vi "SLL DE AI Channel Unit Infomation.vi"(8 "error in (no error)":errorcluster) -> (0 "error out":errorcluster, 3 "Unit Infomation":T2(array[cluster]))   [LabVIEW 2013]
doc: "Copyright © 2005, Soliton Technologies.\nAll rights reserved."
uses:
  Controls/SLL DE DAQ Parameters LV2Global Options.ctl
  Controls/SLL DE List of AI Channel Type.ctl
  Controls/SLL DE Unit Info LV2Global Options.ctl
panel:
  in  "Channel Type":T1
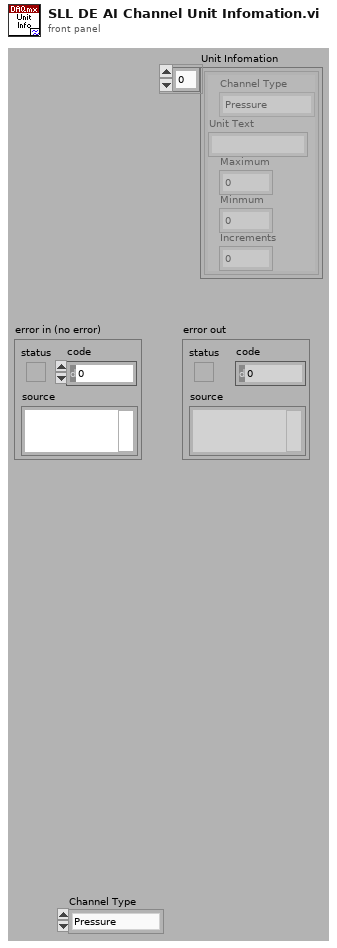
[diagram p1: front panel]
types:
  T1 = typedef "SLL DE List of AI Channel Type.ctl" = enum16{"Pressure", "Flow", "Temperature", "Time Scale", "Voltage", "Current", "Frequency", "Sound", "Speed", "Torque", "Distance", "Channel Type 1", "Channel Type 2", "Channel Type 3"}
  T2 = cluster{"Channel Type":T1, "Unit Text":string, "Maximum":dbl, "Minmum":dbl, "Increments":dbl}[]
  T3 = typedef "SLL DE Unit Info LV2Global Options.ctl" = enum16{"Update Channel Type", "Update Unit Info", "Get Unit Info", "Read"}
  T4 = typedef "SLL DE DAQ Parameters LV2Global Options.ctl" = enum16{"Read", "Write"}
  T5 = typedef "SLL DE DAQ Engine Parameters.ctl" = cluster{"Enable Engines":cluster{"AI Enable":bool, "AO Enable":bool, "DI Enable":bool, "DO Enable":bool}, "DAQ Control Type":cluster{"Analog Input":enum16{"Finite", "Continuous", "Driver"}, "Analog Output":enum16{"Finite", "Continuous", "Driver"}, "Digital Input":enum16{"Finite", "Continuous", "Driver"}, "Digital Output":enum16{"Finite", "Continuous", "Driver"}}, "DAQ Parameters":cluster{"AI Sampling Rate (Samples/Sec)":dbl, "MvgAVG Window Size (# of Points)":i32, "Enable Filter":bool, "Enable MvgAVG":bool, "Circular Buffer Size (Sec)":dbl, "AO Sampling Rate (Samples/Sec)":dbl, "Graph Update Rate (Samples/Sec)":dbl, "File Logging Rate (Samples/Sec)":i32}, "AO Safe Values":cluster{"Analog Outputs Name":T6, "Analog Outputs Safe Value":dbl}[], "DO Safe Values":cluster{"Digital Outputs Name":T7, "Digital Outputs Safe Value":bool}[], "DO Interconnected Lines":cluster{"First DO Line":string, "Second DO Line":string}[], "AI Channels Unit":cluster{"Channel Name":T8, "Channel Type":T1}[], "Units Information":cluster{"Channel Type":T1, "Unit Text":string, "Maximum":dbl, "Minmum":dbl, "Increments":dbl}[]}
  T6 = typedef "SLL DE List of Analog Outputs.ctl" = enum16{"None"}
  T7 = typedef "SLL DE List of Digital Outputs.ctl" = enum16{"STATION1_START TEST", "STATION1_STOP TEST", "STATION1_LIGHT1", "STATION1_LIGHT2", "STATION1_LIGHT3", "STATION1_SELECT_TEST", "STATION2_START TEST", "STATION2_STOP TEST", "STATION2_LIGHT1", "STATION2_LIGHT2", "STATION2_LIGHT3", "STATION2_SELECT_TEST", "STATION3_START TEST", "STATION3_STOP TEST", "STATION3_LIGHT1", "STATION3_LIGHT2", "STATION3_LIGHT3", "STATION3_SELECT_TEST", "STATION4_START TEST", "STATION4_STOP TEST", "STATION4_LIGHT1", "STATION4_LIGHT2", "STATION4_LIGHT3", "STATION4_SELECT_TEST"}
  T8 = typedef "SLL DE List of Analog Inputs.ctl" = enum16{"None"}
  T9 = cluster{"Channel Type":T1, "Unit Text":string, "Maximum":dbl, "Minmum":dbl, "Increments":dbl}
  T10 = cluster{"Channel Type":T1, string, "Maximum":dbl, "Minmum":dbl, "Increments":dbl}
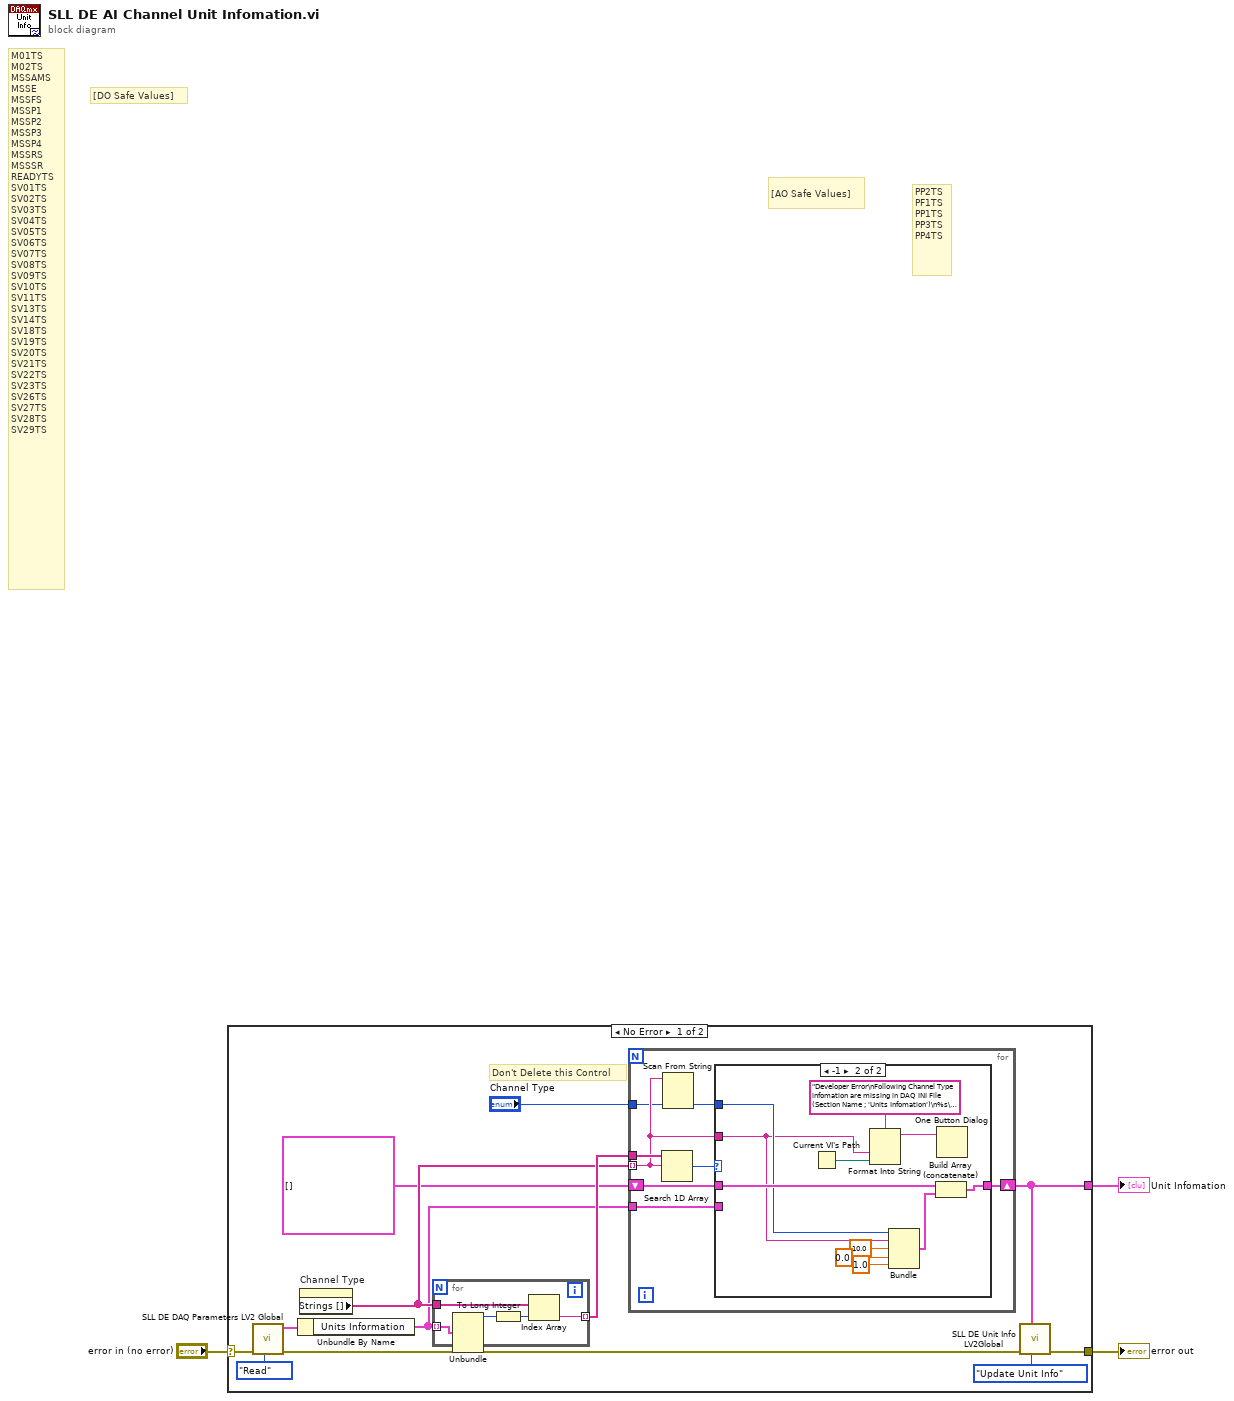
[diagram p0: block diagram]
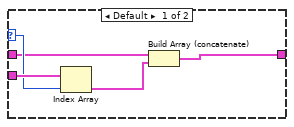
[diagram p2: hidden frame]
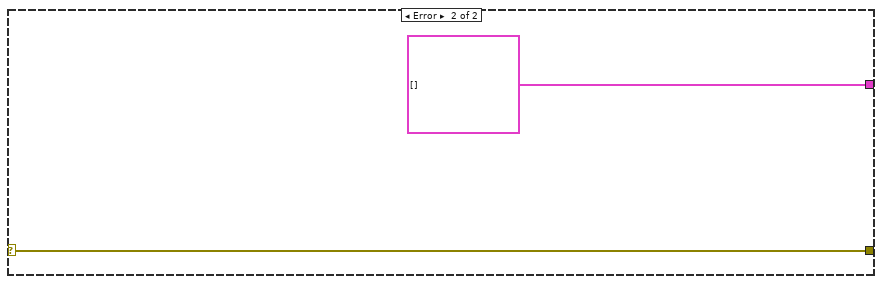
[diagram p3: hidden frame]
diagram:
  # "[DO Safe Values]"
  # "PP2TS\nPF1TS\nPP1TS\nPP3TS\nPP4TS"
  # "[AO Safe Values]"
  # "M01TS\nM02TS\nMSSAMS\nMSSE\nMSSFS\nMSSP1\nMSSP2\nMSSP3\nMSSP4\nMSSRS\nMSSSR\nREADYTS\nSV01TS\nSV02TS\nSV03TS\nSV04TS\nSV05TS\nSV06TS\nSV07TS\nSV08TS\nSV09TS\nSV10TS\nSV11TS\nSV13TS\nSV14TS\nSV18TS\nSV19TS\nSV20TS\nSV21TS\nSV22TS\nSV23TS\nSV26TS\nSV27TS\nSV28TS\nSV29TS"
  n1 = case shown="No Error" "error in (no error)" {
    selector: "error in (no error)" -> [w12 w46]
    tunnel: [w5 w46] -> w2
    tunnel: [w4 T2 []] -> w1
    frame No Error {
      # "Don't Delete this Control"
      n2 = call "SLL DE DAQ Parameters LV2 Global.vi"("Option"=SLL_DE_DAQ_Parameters_LV2Global_Options."Read", "Error in (no error)"=w12) -> ("Error out"=w6:errorcluster, "Global Info"=w14:T5)  [unwired: 8 in]
      n3 = Unbundle By Name(w14) -> ("Units Information"=w9:T2)
      n4 = property on="Channel Type" class="Enum (strict)"() -> ("Strings []"=w10:string[])  [unwired: 2 in, 2 out]
      n5 = for {
        tunnel: w9 -> [w20] mode=indexing
        tunnel: w10 -> [w17]
        tunnel: [w16] -> w11 mode=indexing
        n6 = Unbundle(w20) -> ("Channel Type"=w19:T1)  [unwired: 4 out]
        n7 = To Long Integer(number=w19) -> (32bit integer=w18:i32)
        n8 = Index Array(array=w17, index=w18) -> (element=w16:string)
      }
      n9 = for {
        tunnel: w11 -> [w28]
        tunnel: w10 -> [w24] mode=indexing
        shift-right: [w26] -> w4
        shift-left: T2 [] -> [w25]
        tunnel: "Channel Type" -> [w23]
        tunnel: w9 -> [w22]
        n10 = Search 1D Array(1D array=w28, element=w24) -> (index of element=w27:i32)  [unwired: 1 in]
        n11 = Scan From String(input string=w24, default 1=w23) -> (output 1=w21:T1)  [unwired: 3 in, 3 out]
        n12 = case shown="-1" w27 {
          selector: w27 -> [w32 _]
          tunnel: w22 -> [w33 _]
          tunnel: [w31 w43] -> w26
          tunnel: w25 -> [w30 w44]
          tunnel: w24 -> [_ w34]
          tunnel: w21 -> [_ w40]
          frame Default {
            n13 = Index Array(array=w33, index=w32) -> (element=w29:T9)
            n14 = Build Array (concatenate)(w30, w29) -> (w31:T2)
          }
          frame -1 {
            n15 = Current VI's Path() -> (path=w42:path)
            n16 = Format Into String(format string="Developer Error\nFollowing Channel Type infomation are missing in DAQ INI File (Section Name ; 'Units Infomation')\n%s\n%s" ("message"), w34, w42) -> (resulting string=w41:string)  [unwired: 2 in, 1 out]
            n17 = Bundle("Channel Type"=w40, w34, "Maximum"=10.0, "Minmum"=0.0, "Increments"=1.0) -> (w39:T10)  [unwired: 1 in]
            n18 = Build Array (concatenate)(w44, w39) -> (w43:T2)
            n19 = One Button Dialog(message=w41) -> ()  [unwired: 1 in, 1 out]
          }
        }
      }
      n20 = call "SLL DE Unit Info LV2Global.vi"("Option"=SLL_DE_Unit_Info_LV2Global_Options."Update Unit Info", "Units Information"=w4, "Error in (no error)"=w6) -> ("Error out"=w5:errorcluster)  [unwired: 6 in, 2 out]
    }
    frame Error {
    }
  }
  "error out" <- w2
  "Unit Infomation" <- w1
